vi "DAQmx - FGV(V)_SubVIs-某型振动实验台测试系统.vi"(7 "Operation":T8, 8 "Error In":errorcluster, 11 "Task Info":T2={"Accele Task"=[], "Simulate"=FALSE, "采样率"={"AISampleRate"=10123, "CouplingType"=10000, "Butter"=1000}, "Trig"={"PreTrigCNT"=0, "TriggerMode"=enum."中间触发", "TriggerSource"=enum."软件触发", "ATRTriggerChannel"=enum."通道0", "TriggerDir"=enum."下降沿触发", "TrigLevelVolt"=0.0, "bAvailableTrig"=FALSE}, "clock"={"EN"=FALSE, "clocksource"=enum."内部时钟", "outclocksource"=enum."Trig0"}, "delay(S)"=0.0} {"采样率"."CouplingType" items=["直流耦合", "交流耦合"]}) -> (0 "Error Out":errorcluster, 1 "Data":waveform(dbl)[](array[waveform]), 2 "task done?":bool, 3 "task OUT":T1={"Task Info"={"Accele Task"=[], "Simulate"=FALSE, "采样率"={"AISampleRate"=10123, "CouplingType"=10000, "Butter"=1000}, "Trig"={"PreTrigCNT"=0, "TriggerMode"=enum."中间触发", "TriggerSource"=enum."软件触发", "ATRTriggerChannel"=enum."通道0", "TriggerDir"=enum."下降沿触发", "TrigLevelVolt"=0.0, "bAvailableTrig"=FALSE}, "clock"={"EN"=FALSE, "clocksource"=enum."内部时钟", "outclocksource"=enum."Trig0"}, "delay(S)"=0.0}, "datain"={"nSegmentCount"=0, "chaneldataSize"=8192, "t0 in"=timestamp(0 s since 1904-01-01), "nsegmentsize"=0, "chanelcouter"=0}, "times"=0.0, "timer"=[], "\nen"=FALSE} {"Task Info"."采样率"."CouplingType" items=["直流耦合", "交流耦合"]}, 5 "pDMAStatus out":i32[](array[numeric]))   [LabVIEW 2009]
uses:
  Ctrls/Enum DAQmx - FGV(V)_Ctrls-某型振动实验台测试系统.ctl
  Ctrls/Acceleration Channel Config_Ctrls-某型振动实验台测试系统.ctl
  Ctrls/Sample Information.ctl
  Ctrls/Task Info.ctl
  Ctrls/Trig.ctl
  Ctrls/clock.ctl
  Ctrls/DATA info.ctl
  Ctrls/task.ctl
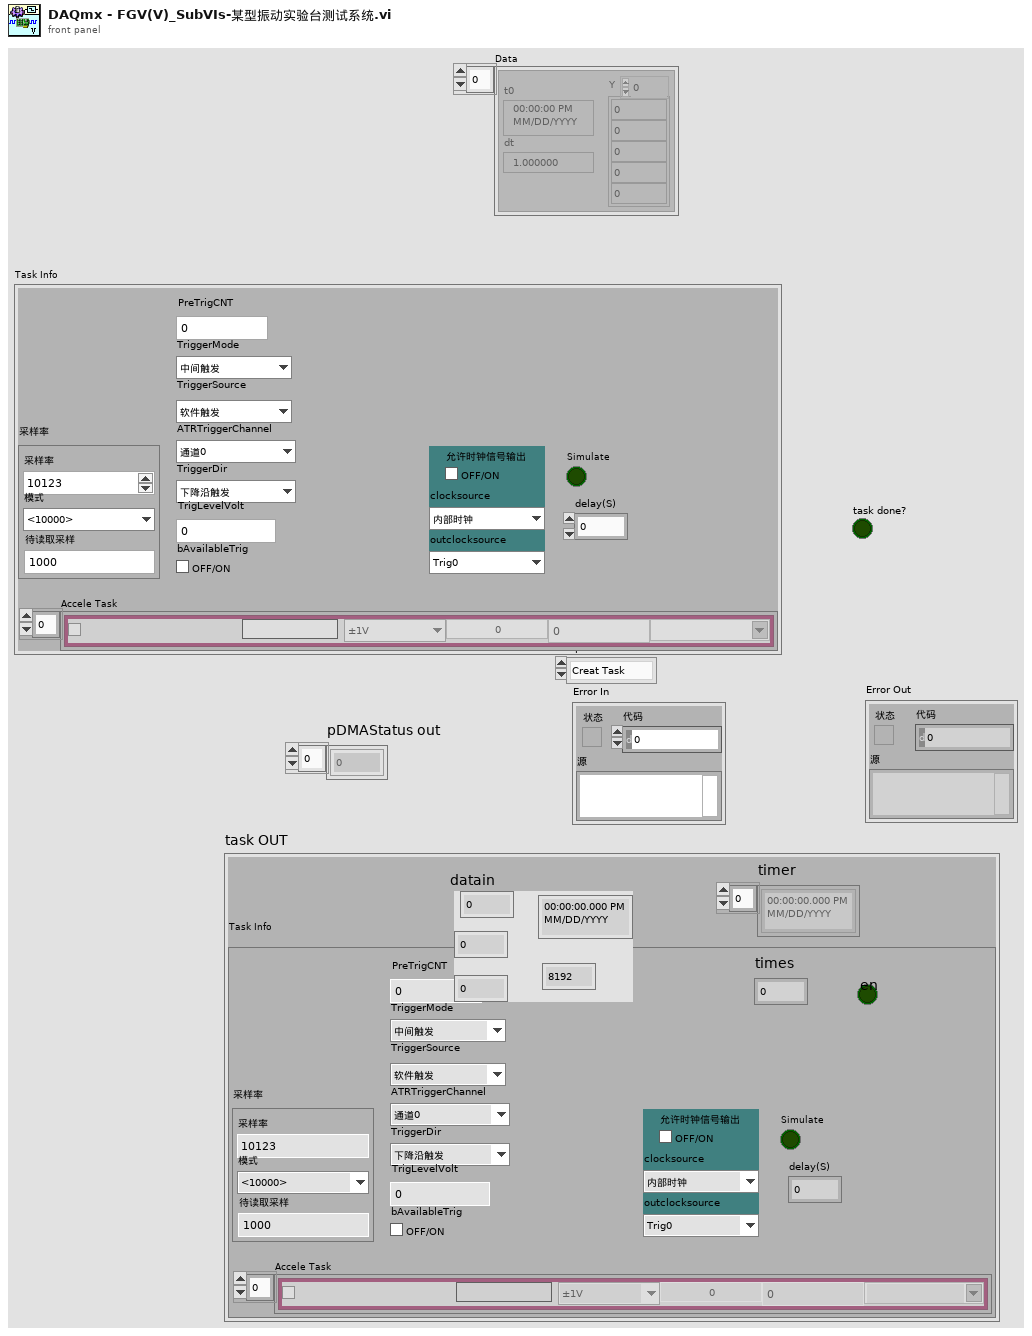
[diagram p1: front panel]
types:
  T1 = typedef "task.ctl" = cluster{"Task Info":T2, "datain":T7, "times":dbl, "timer":timestamp[], "\nen":bool}
  T2 = typedef "Task Info.ctl" = cluster{"Accele Task":T3[], "Simulate":bool, "采样率":T4, "Trig":T5, "clock":T6, "delay(S)":dbl}
  T3 = typedef "Acceleration Channel Config_Ctrls-某型振动实验台测试系统.ctl" = cluster{"Enable":bool, "Name":string, "range":enum16{"±1V", "±5V"}, "SensValue":dbl, "PhysicalName":string, "off":dbl, "Sensunits":string}
  T4 = typedef "Sample Information.ctl" = cluster{"AISampleRate":i32, "CouplingType":i32, "Butter":i32}
  T5 = typedef "Trig.ctl" = cluster{"PreTrigCNT":i32, "TriggerMode":enum16{"中间触发", "后触发", "预触发", "硬件延时触发"}, "TriggerSource":enum16{"软件触发", "DTR信号源", "ATR信号源", "Triger信号触发"}, "ATRTriggerChannel":enum16{"通道0", "通道1", "通道2", "通道3"}, "TriggerDir":enum16{"下降沿触发", "上升沿触发", "上下边没均触发"}, "TrigLevelVolt":sgl, "bAvailableTrig":bool}
  T6 = typedef "clock.ctl" = cluster{"EN":bool, "clocksource":enum16{"内部时钟", "外部时钟"}, "outclocksource":enum16{"Trig0", "Trig1", "Trig2", "Trig3", "Trig4", "Trig5", "Trig6", "Trig7", "PXI_STAR"}}
  T7 = typedef "DATA info.ctl" = cluster{"nSegmentCount":i32, "chaneldataSize":i32, "t0 in":timestamp, "nsegmentsize":i32, "chanelcouter":i32}
  T8 = typedef "Enum DAQmx - FGV(V)_Ctrls-某型振动实验台测试系统.ctl" = enum16{"Creat Task", "Start Task", "Read Data", "Check Task", "Stop Task", "Clear Task"}
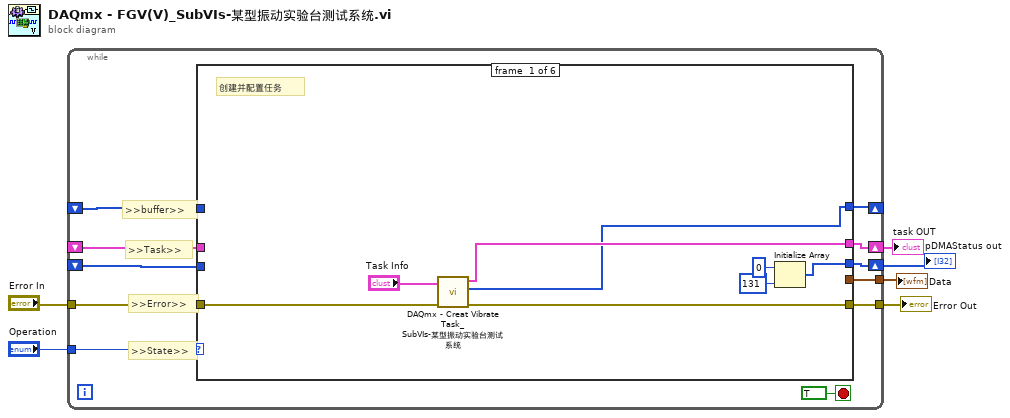
[diagram p0: block diagram]
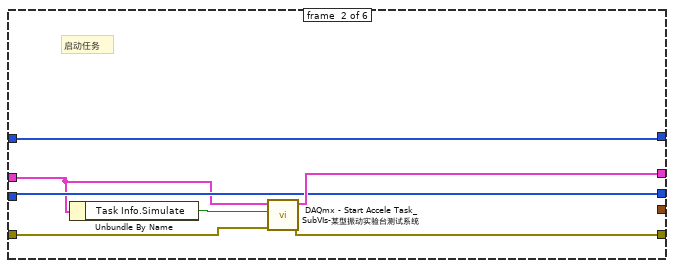
[diagram p2: hidden frame]
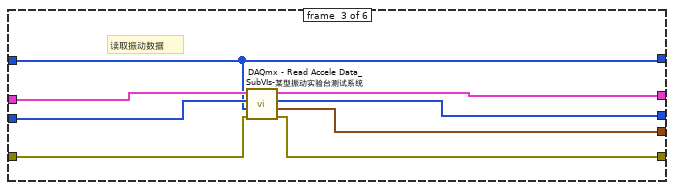
[diagram p3: hidden frame]
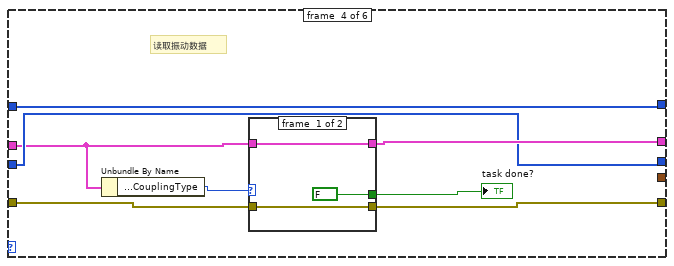
[diagram p4: hidden frame]
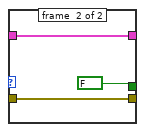
[diagram p5: hidden frame]
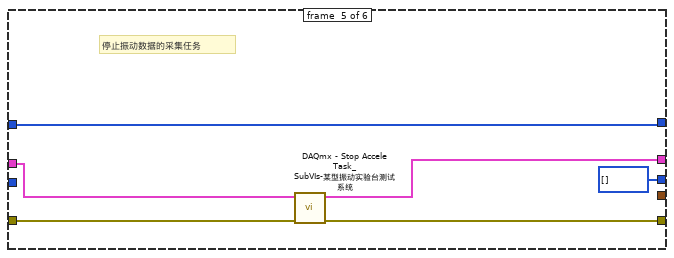
[diagram p6: hidden frame]
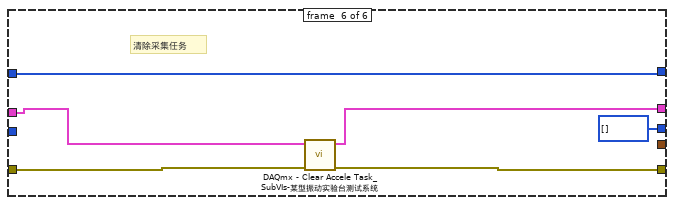
[diagram p7: hidden frame]
diagram:
  n1 = while {
    tunnel: "Operation" -> [w17]
    shift-right: [w13] -> w3
    shift-left: _ -> [w15]
    tunnel: "Error In" -> [w11]
    tunnel: [w14] -> w4
    shift-right: [w12] -> _
    shift-left: _ -> [w10]
    shift-right: [w9] -> w1
    shift-left: _ -> [w8]
    tunnel: [w7] -> w2
    stop <- TRUE stop-if-true
    # ">>buffer>>"
    # ">>State>>"
    # ">>Error>>"
    # ">>Task>>"
    n2 = case shown="\"Start Task\"" w17 {
      tunnel: w15 -> [_ w27 w39 w41 w56 w62]
      tunnel: w11 -> [w20 w32 w33 w46 w59 w65]
      tunnel: [w24 w31 w40 w47 w58 w64] -> w14
      tunnel: [w25 w30 w38 w48 w55 w61] -> w13
      tunnel: [w18 w29 w35 w45 w60 w66] -> w12
      tunnel: w10 -> [_ w29 w35 w45 w60 w66]
      tunnel: [w23 w28 w37 w42 i32[] [] ("pDMAStatus out") i32[] [] ("pDMAStatus out")] -> w9
      tunnel: w8 -> [_ w28 w36 w42 _ _]
      tunnel: [_ _ w34 _ _ _] -> w7
      frame #0 {
        # "创建并配置任务"
        n3 = call "DAQmx - Creat Vibrate Task_SubVIs-某型振动实验台测试系统.vi"("Error In"=w20, "Task info"="Task Info") -> ("error out"=w24:errorcluster, "ADBuffer"=w18:u16[], "task out"=w25:T1)  [unwired: 7 out]
        n4 = Initialize Array(0 ("element"), 131 ("dimension size")) -> (w23:i32[])
      }
      frame #1 {
        # "启动任务"
        n5 = Unbundle By Name(w27) -> ("Task Info.Simulate"=w26:bool)
        n6 = call "DAQmx - Start Accele Task_SubVIs-某型振动实验台测试系统.vi"("Error In"=w32, "Simulate"=w26, "task"=w27) -> ("Error out"=w31:errorcluster, "task out"=w30:T1)  [unwired: 7 out]
      }
      frame #2 {
        # "读取振动数据"
        n7 = call "DAQmx - Read Accele Data_SubVIs-某型振动实验台测试系统.vi"("Error In"=w33, "Buffer"=w35, "pDMAStatus"=w36, "task in"=w39) -> ("Error Out"=w40:errorcluster, "Data"=w34:waveform(dbl)[], "pDMAStatus out"=w37:i32[], "task out"=w38:T1)  [unwired: 2 in, 2 out]
      }
      frame #3 {
        # "读取振动数据"
        n8 = Unbundle By Name(w41) -> ("Task Info.采样率.CouplingType"=w44:i32)
        n9 = case shown="10178" w44 {
          tunnel: w41 -> [w51 w53]
          tunnel: [w51 w53] -> w48
          tunnel: [w50 w54] -> w47
          tunnel: w46 -> [w50 w54]
          tunnel: [FALSE FALSE] -> w43
          frame #0 {
          }
          frame #1 {
          }
        }
        "task done?" <- w43
      }
      frame #4 {
        # "停止振动数据的采集任务"
        n10 = call "DAQmx - Stop Accele Task_SubVIs-某型振动实验台测试系统.vi"("Error In"=w59, "task  IN"=w56) -> ("Error Out"=w58:errorcluster, "task OUT"=w55:T1)  [unwired: 4 in, 4 out]
      }
      frame #5 {
        # "清除采集任务"
        n11 = call "DAQmx - Clear Accele Task_SubVIs-某型振动实验台测试系统.vi"("Error In"=w65, "task IN"=w62) -> ("Error Out"=w64:errorcluster, "task OUT"=w61:T1)  [unwired: 3 in, 5 out]
      }
    }
  }
  "Error Out" <- w4
  "task OUT" <- w3
  "Data" <- w2
  "pDMAStatus out" <- w1
